vi "PS_MEASURE_V-I_Ary.vi"(0 "VISA resource name":refnum<visa-resource-name>, 1 "SEL_PS":string(combo), 11 "error in (no error)":errorcluster {"code" format="%.0x"}, 12 "Array 2":bool[](array[boolean])=[TRUE, FALSE, FALSE, FALSE], 14 "Measurement Type (1: Voltage)":i32(ring) items=["Current", "Voltage"]) -> (4 "VISA resource name out":refnum<visa-resource-name>, 6 "Array":dbl[](array[numeric]), 15 "error out":errorcluster {"code" format="%.0x"})   [LabVIEW 2018]
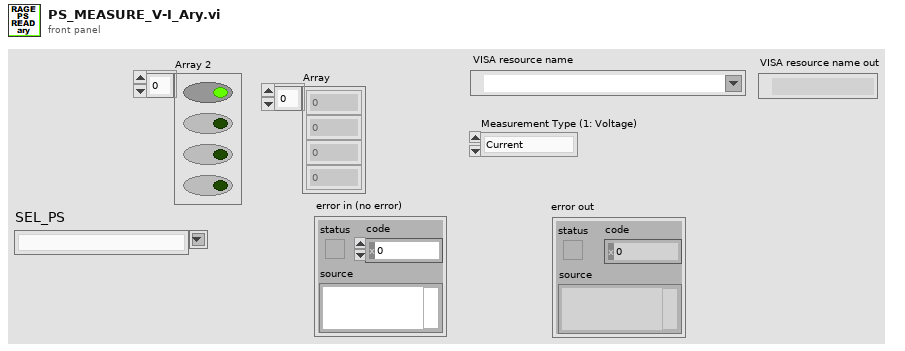
[diagram p1: front panel]
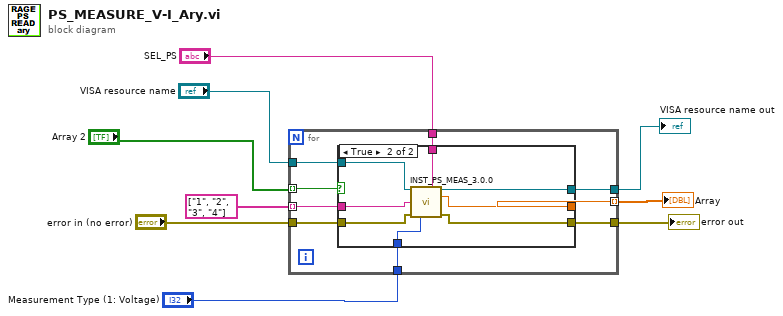
[diagram p0: block diagram]
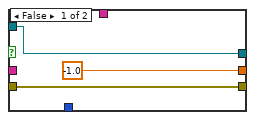
[diagram p2: hidden frame]
diagram:
  n1 = for {
    tunnel: string[] ["1", "2", "3", "4"] -> [w18] mode=indexing
    tunnel: "error in (no error)" -> [w17]
    tunnel: [w16] -> w7
    tunnel: "Array 2" -> [w15] mode=indexing
    tunnel: [w14] -> w5 mode=indexing
    tunnel: "VISA resource name" -> [w13]
    tunnel: "Measurement Type (1: Voltage)" -> [w12]
    tunnel: [w11] -> w2
    tunnel: "SEL_PS" -> [w10]
    n2 = case shown="True" w15 {
      tunnel: w18 -> [_ w23]
      tunnel: w17 -> [w21 w29]
      tunnel: [w21 w25] -> w16
      tunnel: [-1.0 ("Measurement") w26] -> w14
      tunnel: w13 -> [w19 w28]
      tunnel: w12 -> [_ w24]
      tunnel: [w19 w27] -> w11
      tunnel: w10 -> [_ w22]
      frame False {
      }
      frame True {
        n3 = call "INST_PS_MEAS_3.0.0.vi"("VISA session"=w28, "SEL_PS"=w22, "Channel Name (1)"=w23, "error in (no error)"=w29, "Measurement Type (1: Voltage)"=w24) -> ("dup VISA session"=w27:refnum<visa-resource-name>, "Measurement"=w26:dbl, "error out"=w25:errorcluster)  [unwired: 7 in, 1 out]
      }
    }
  }
  "error out" <- w7
  "Array" <- w5
  "VISA resource name out" <- w2
